vi "Valid VI Reference.vi"(1 "VI Refnum":refnum<vi>) -> (8 "Valid?":bool)   [LabVIEW 2014]
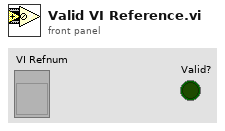
[diagram p1: front panel]
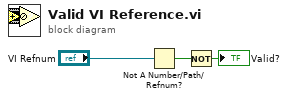
[diagram p0: block diagram]
diagram:
  n1 = Not A Number/Path/Refnum?(number/path/refnum="VI Refnum") -> (NaN/Path/Refnum?=w3:bool)
  n2 = Not(x=w3) -> (.not. x?=→"Valid?":bool)
